vi "_016.vi"() -> ()   [LabVIEW 2024]
panel:
  out "n--":i32[](array[numeric])
  out "n++":i32[](array[numeric])
  out "Tables":dbl[](array[numeric])
  out "Odd":dbl[](array[numeric])
  out "Even":dbl[](array[numeric])
  # "For Loop (Dfrnt opearation's)"
  # "Separate odd & even :"
  # "Tables :"
  # "Print no. in Ascending"
  # "& Descending :"
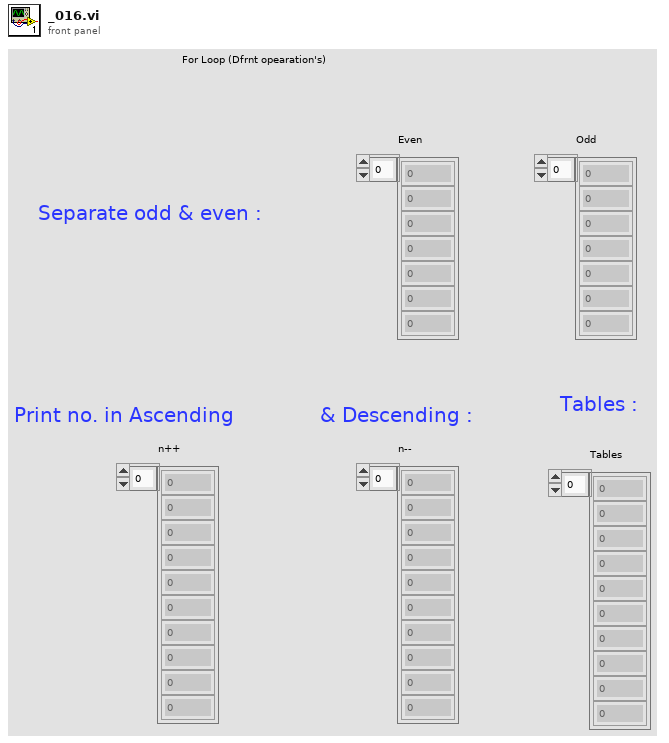
[diagram p1: front panel]
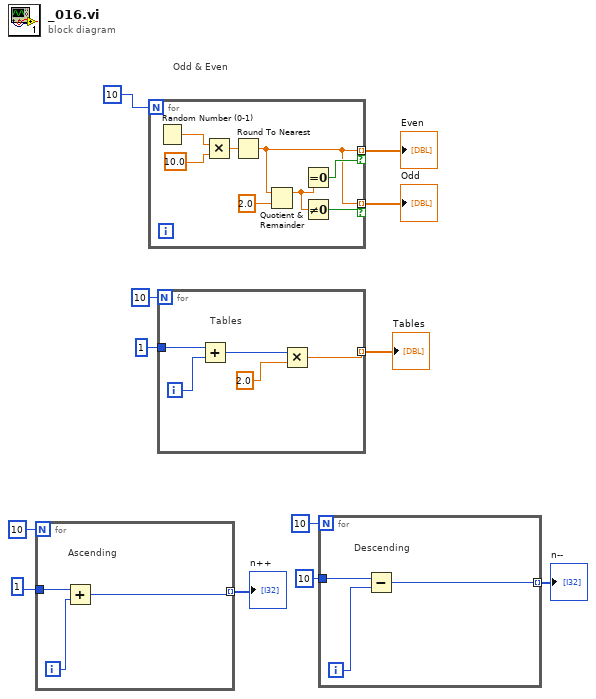
[diagram p0: block diagram]
diagram:
  # "Odd & Even"
  n1 = for {
    N: 10 -> [_]
    tunnel: 1 -> [w15]
    tunnel: [w13] -> w4 mode=indexing
    i -> [w14]
    # "Ascending"
    n2 = Add(x=w15, y=w14) -> (x+y=w13:i32)
  }
  "n++" <- w4
  n3 = for {
    N: 10 -> [_]
    tunnel: [w16] -> w11 mode=indexing if=w19
    tunnel: [w16] -> w10 mode=indexing if=w18
    n4 = Random Number (0-1)() -> (number: 0 to 1=w23:dbl)
    n5 = Multiply(x=w23, y=10.0) -> (x*y=w22:dbl)
    n6 = Round To Nearest(number=w22) -> (nearest integer value=w16:dbl)
    n7 = Quotient & Remainder(x=w16, y=2.0) -> (x-y*floor(x/y)=w20:dbl)  [unwired: 1 out]
    n8 = Equal To 0?(x=w20) -> (x = 0?=w19:bool)
    n9 = Not Equal To 0?(x=w20) -> (x != 0?=w18:bool)
  }
  "Even" <- w11
  "Odd" <- w10
  n10 = for {
    N: 10 -> [_]
    tunnel: 1 -> [w27]
    tunnel: [w24] -> w7 mode=indexing
    i -> [w28]
    # "Tables"
    n11 = Add(x=w27, y=w28) -> (x+y=w25:i32)
    n12 = Multiply(x=w25, y=2.0) -> (x*y=w24:dbl)
  }
  "Tables" <- w7
  n13 = for {
    N: 10 -> [_]
    tunnel: 10 -> [w31]
    tunnel: [w29] -> w1 mode=indexing
    i -> [w30]
    # "Descending"
    n14 = Subtract(x=w31, y=w30) -> (x-y=w29:i32)
  }
  "n--" <- w1
